vi "putApple_subVI.vi"(9 "Field Width":i32, 10 "Field Height":i32, 11 "Snake Field in":u32[][](array[numeric])) -> (3 "Snake Field out":u32[][](array[numeric]))   [LabVIEW 2020]
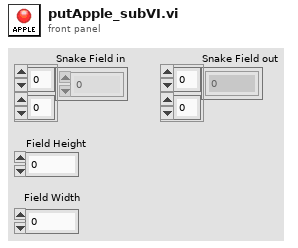
[diagram p1: front panel]
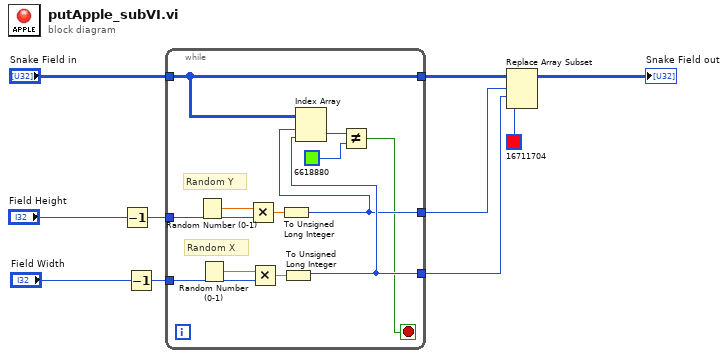
[diagram p0: block diagram]
diagram:
  n1 = Decrement(x="Field Height") -> (x-1=w5:i32)
  n2 = Decrement(x="Field Width") -> (x-1=w3:i32)
  n3 = while {
    tunnel: [w14] -> w10
    tunnel: [w15] -> w9
    tunnel: w5 -> [w18]
    tunnel: w3 -> [w17]
    tunnel: "Snake Field in" -> [w16]
    tunnel: [w16] -> w1
    stop <- w11 stop-if-true
    # "Random Y"
    # "Random X"
    n4 = Random Number (0-1)() -> (number: 0 to 1=w22:dbl)
    n5 = Random Number (0-1)() -> (number: 0 to 1=w19:dbl)
    n6 = Multiply(x=w22, y=w18) -> (x*y=w21:dbl)
    n7 = Multiply(x=w19, y=w17) -> (x*y=w20:dbl)
    n8 = To Unsigned Long Integer(number=w21) -> (unsigned 32bit integer=w14:u32)
    n9 = To Unsigned Long Integer(number=w20) -> (unsigned 32bit integer=w15:u32)
    n10 = Index Array(array=w16, index (row)=w14, index (col)=w15) -> (element=w13:u32)
    n11 = Not Equal?(x=w13, y=u32 6618880 ("Color Box")) -> (x != y?=w11:bool)
  }
  n12 = Replace Array Subset(array=w1, new element=u32 16711704 ("Color Box"), index (row)=w10, index (col)=w9) -> (→"Snake Field out":u32[][])
